vi "Motic Set Flip.vi"(8 "error in (no error)":errorcluster, 10 "b":bool, 11 "camera":i32) -> (0 "error out":errorcluster, 3 "camera out":i32)   [LabVIEW 2012, in "MoticApi.lvlib"]
doc: "MOTICAPI bool Motic_SetFlip(MUCam_Handle camera, bool b);"
uses:
  MoticApi.lvlib
  MoticApi.dll
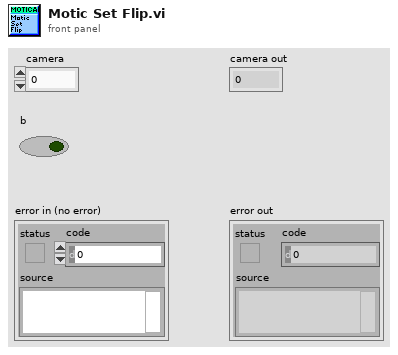
[diagram p1: front panel]
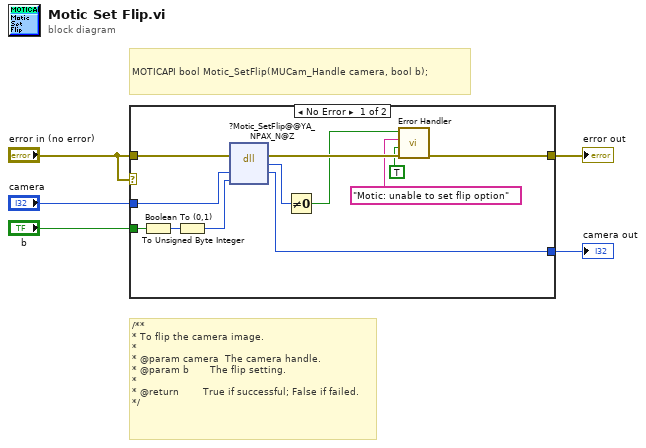
[diagram p0: block diagram]
diagram:
  # "/**\n* To flip the camera image.\n*\n* @param camera  The camera handle.\n* @param b       The flip setting.\n*\n* @return        True if successful; False if failed.\n*/"
  # "MOTICAPI bool Motic_SetFlip(MUCam_Handle camera, bool b);"
  n1 = case shown="No Error" "error in (no error)" {
    tunnel: "camera" -> [w16 w18]
    tunnel: [w15 w18] -> w4
    tunnel: "b" -> [w14 _]
    tunnel: "error in (no error)" -> [w13 w19]
    tunnel: [w11 w19] -> w2
    frame No Error {
      n2 = Boolean To (0,1)(Boolean=w14) -> (0, 1=w8:i16)
      n3 = To Unsigned Byte Integer(number=w8) -> (unsigned 8bit integer=w7:u8)
      n4 = dll-call lib="C:/Users/TTS-Digital/Desktop/MoticApi/MoticApi_git/MoticApi/MoticApi.*" fn="?Motic_SetFlip@@YA_NPAX_N@Z"(error in=w13, "camera"=w16, "b"=w7) -> (error out=w12:errorcluster, w17:u8, "camera"=w15:i32)  [unwired: 3 in, 1 out]
      n5 = Not Equal To 0?(x=w17) -> (x != 0?=w10:bool)
      n6 = call "Error Handler.vi"("error in (no error)"=w12, "Is warning?"=TRUE, "Error message"="Motic: unable to set flip option", "Function return"=w10) -> ("error out"=w11:errorcluster)  [unwired: 7 in]
    }
    frame Error {
    }
  }
  "camera out" <- w4
  "error out" <- w2
